vi "setAxisGrid.vi"(7 "Grids":T2, 8 "polarGridAngle":dbl, 9 "Axis":T1="x", 11 "String in":string) -> (2 "command":string, 3 "String out":string)   [LabVIEW 2012]
uses:
  grids.ctl
  axisName.ctl
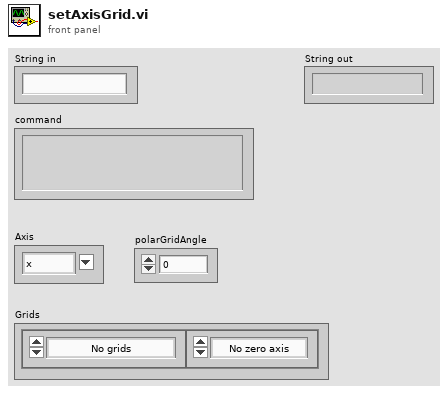
[diagram p1: front panel]
types:
  T1 = typedef "axisName.ctl" = string
  T2 = typedef "grids.ctl" = cluster{"Gridlines":enum16{"No grids", "Major grid", "Minor grid", "Major and Minor"}, "Zeroaxis":enum16{"No zero axis", "Show zero axis"}}
  T3 = enum16{"No grids", "Major grid", "Minor grid", "Major and Minor"}
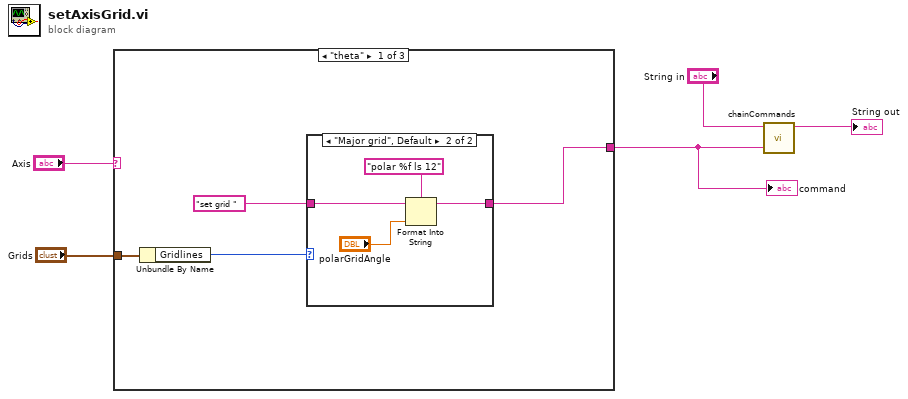
[diagram p0: block diagram]
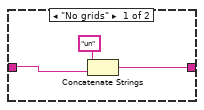
[diagram p2: hidden frame]
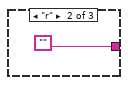
[diagram p3: hidden frame]
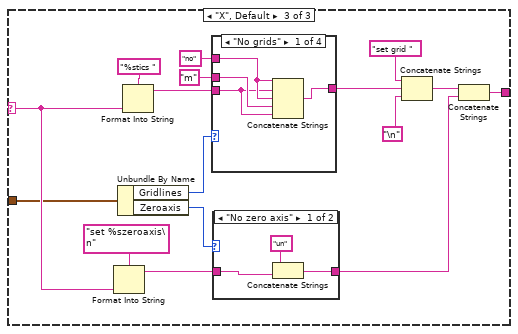
[diagram p4: hidden frame]
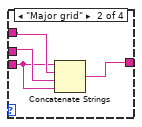
[diagram p6: hidden frame]
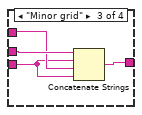
[diagram p7: hidden frame]
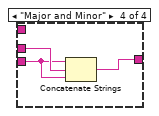
[diagram p8: hidden frame]
diagram:
  n1 = case shown="\"theta\"" "Axis" {
    selector: "Axis" -> [_ _ w19]
    tunnel: [w9 "" w31] -> w3
    tunnel: "Grids" -> [w8 _ w18]
    frame "theta" {
      n2 = Unbundle By Name(w8) -> ("Gridlines"=w6:T3)
      n3 = case shown="\"Major grid\", Default" w6 {
        tunnel: [w12 w14] -> w9
        tunnel: "set grid " ("initial string") -> [w11 w13]
        frame "No grids" {
          n4 = Concatenate Strings("un" ("string"), w11) -> (w12:string)
        }
        frame "Major grid", Default {
          n5 = Format Into String(format string="polar %f ls 12", initial string=w13, "polarGridAngle") -> (resulting string=w14:string)  [unwired: 1 in, 1 out]
        }
      }
    }
    frame "r" {
    }
    frame "X", Default {
      n6 = Format Into String(format string="set %szeroaxis\n", w19) -> (resulting string=w20:string)  [unwired: 2 in, 1 out]
      n7 = Unbundle By Name(w18) -> ("Gridlines"=w29:T3, "Zeroaxis"=w28:enum16{"No zero axis", "Show zero axis"})
      n8 = Format Into String(format string="%stics ", w19) -> (resulting string=w25:string)  [unwired: 2 in, 1 out]
      n9 = case shown="\"No grids\"" w29 {
        tunnel: [w41 w45 w49 w50] -> w33
        tunnel: w25 -> [w38 w42 w46 w51]
        tunnel: "no" ("format string") -> [w40 w44 w47 _]
        tunnel: "m" ("format string") -> [w39 w43 w48 w52]
        frame "No grids" {
          n10 = Concatenate Strings(w40, w38, w40, w39, w38) -> (w41:string)
        }
        frame "Major grid" {
          n11 = Concatenate Strings(w42, w44, w43, w42) -> (w45:string)
        }
        frame "Minor grid" {
          n12 = Concatenate Strings(w48, w46, w47, w46) -> (w49:string)
        }
        frame "Major and Minor" {
          n13 = Concatenate Strings(w51, w52, w51) -> (w50:string)
        }
      }
      n14 = case shown="\"No zero axis\"" w28 {
        tunnel: [w36 w37] -> w30
        tunnel: w20 -> [w35 w37]
        frame "No zero axis" {
          n15 = Concatenate Strings("un", w35) -> (w36:string)
        }
        frame "Show zero axis" {
        }
      }
      n16 = Concatenate Strings("set grid ", w33, "\n") -> (w32:string)
      n17 = Concatenate Strings(w32, w30) -> (w31:string)
    }
  }
  "command" <- w3
  n18 = call "chainCommands.vi"("Command"=w3, "StringIn"="String in") -> ("StringOut"=→"String out":string)  [unwired: 9 in]
